vi "Draw Sky.vi"(9 "draw options":T1={"Text Color"=16777238, "Wing Color"=16751616, "Dial Outline Color"=13816530, "Sky Color"=3381759, "Ground Color"=8213043, "Horizon Line Color"=16777225, "Outline Color"=0, "Dial Background Color"=5987163, "Draw Wings"=TRUE, "Draw Text"=TRUE, "Font Name"="Helvetica", "Angle units"=enum."Radians"}, 10 "draw area state":T3, 11 "picture in":picture) -> (3 "picture out":picture)   [LabVIEW 2017, in "NI_Robotics_Attitude Picture.lvlib"]
uses:
  <vilib>/robotics/Controls/Attitude Indicator/Attitude Picture/NI_Robotics_Attitude Picture.lvlib
  <vilib>/robotics/Controls/Attitude Indicator/Attitude Picture/Draw Area State.ctl
  <vilib>/Utility/miscctls.llb/LVBoundsTypeDef.ctl
  <vilib>/robotics/Controls/Attitude Indicator/Attitude Picture/Draw Options.ctl
  <vilib>/robotics/Controls/Utilities/Angle Units.ctl
  <vilib>/robotics/Controls/Utilities/NI_Robotics_Control Utilities.lvlib
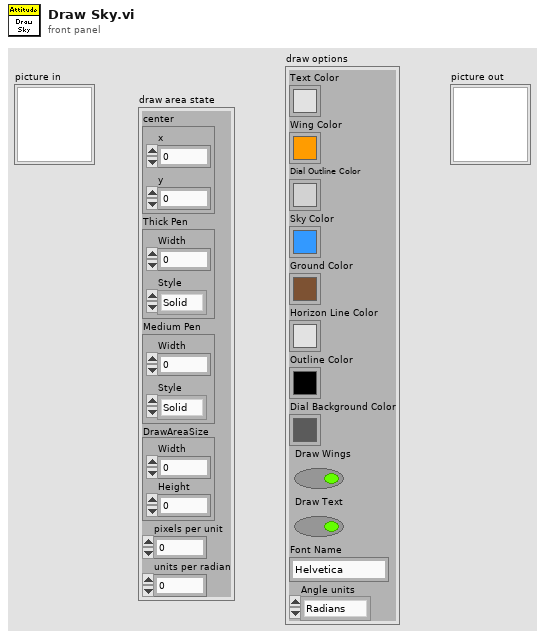
[diagram p1: front panel]
types:
  T1 = typedef "NI_Robotics_Attitude Picture.lvlib/Draw Options.ctl" = cluster{"Text Color":u32, "Wing Color":u32, "Dial Outline Color":u32, "Sky Color":u32, "Ground Color":u32, "Horizon Line Color":u32, "Outline Color":u32, "Dial Background Color":u32, "Draw Wings":bool, "Draw Text":bool, "Font Name":string, "Angle units":T2}
  T2 = typedef "NI_Robotics_Control Utilities.lvlib/Angle Units.ctl" = enum16{"Radians", "Degrees"}
  T3 = typedef "NI_Robotics_Attitude Picture.lvlib/Draw Area State.ctl" = cluster{"center":cluster{"x":i16, "y":i16}, "Thick Pen":cluster{"Width":u16, "Style":enum32{"Solid", "Dash", "Dot", "DashDot", "DashDotDot"}}, "Medium Pen":cluster{"Width":u16, "Style":enum32{"Solid", "Dash", "Dot", "DashDot", "DashDotDot"}}, "DrawAreaSize":T4, "pixels per unit":dbl, "units per radian":dbl}
  T4 = typedef "LVBoundsTypeDef.ctl" = cluster{"Width":u32, "Height":u32}
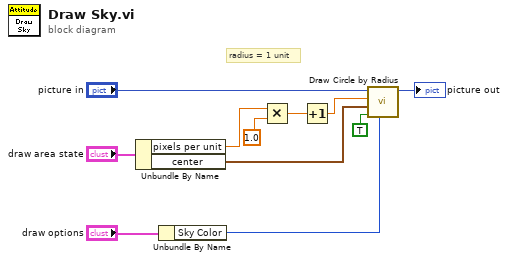
[diagram p0: block diagram]
diagram:
  # "radius = 1 unit"
  n1 = Unbundle By Name("draw area state") -> ("pixels per unit"=w7:dbl, "center"=w5:cluster{"x":i16, "y":i16})
  n2 = Unbundle By Name("draw options") -> ("Sky Color"=w3:u32)
  n3 = Multiply(x=w7, y=1.0) -> (x*y=w2:dbl)
  n4 = Increment(x=w2) -> (x+1=w1:dbl)
  n5 = call <vilib>:"Draw Circle by Radius.vi"("color(black)"=w3, "fill?(F)"=TRUE, "pixel center"=w5, "radius"=w1, "picture"="picture in") -> ("new picture"=→"picture out":picture)  [unwired: 6 in]
